vi "get_instances.vi"(6 "id (unnamed)":string, 8 "error in (no error)":errorcluster, 10 "Base Class (LabVIEW Object)":refnum<class>, 11 "Lookup Service in":refnum<class "Lookup Service.lvclass">) -> (0 "error out":errorcluster, 2 "instances":set{refnum<data-value>}(c389), 3 "Lookup Service out":refnum<class "Lookup Service.lvclass">)   [LabVIEW 2019, in "Lookup API.lvlib" / "Lookup Service.lvclass"]
uses:
  Lookup Service.lvclass
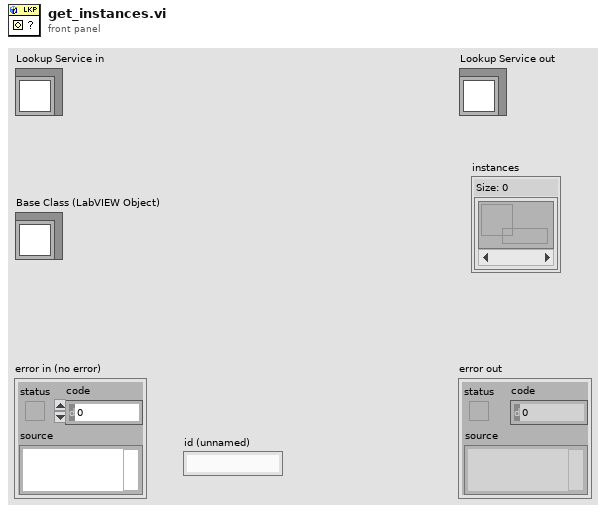
[diagram p1: front panel]
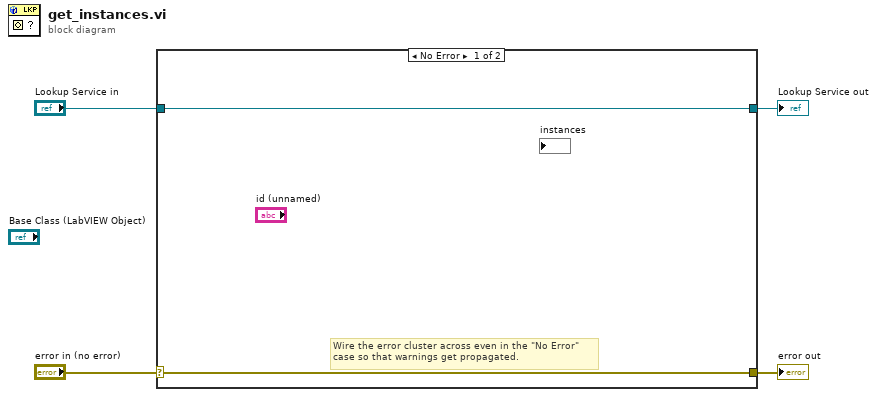
[diagram p0: block diagram]
diagram:
  n1 = case shown="No Error" "error in (no error)" {
    selector: "error in (no error)" -> [w5 w8]
    tunnel: [w5 w8] -> w3
    tunnel: [w6 w7] -> w1
    tunnel: "Lookup Service in" -> [w6 w7]
    frame No Error {
      # "Wire the error cluster across even in the \"No Error\"\ncase so that warnings get propagated."
    }
    frame Error {
    }
  }
  "error out" <- w3
  "Lookup Service out" <- w1
